vi "Exclude Zero Noise.vi"(7 "Counter in":dbl, 9 "RBF Weights in":dbl[](array[numeric]), 11 "RBF Weights previous in":dbl[](array[numeric])) -> (2 "RBF Weights out":dbl[](array[numeric]), 5 "Counter out":dbl)   [LabVIEW 2021]
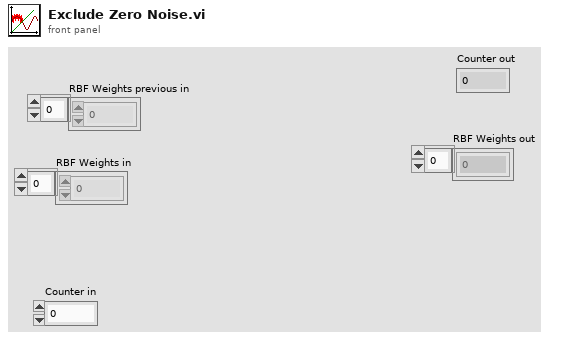
[diagram p1: front panel]
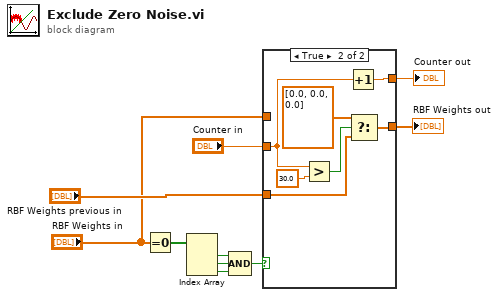
[diagram p0: block diagram]
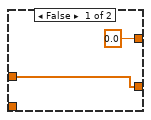
[diagram p2: hidden frame]
diagram:
  n1 = Equal To 0?(x="RBF Weights in") -> (x = 0?=w10:bool[])
  n2 = Index Array(array=w10) -> (element #1=w9:bool, element #2=w8:bool, element #3=w7:bool)  [unwired: 3 in]
  n3 = Compound Arithmetic op=AND(w9, w8, w7) -> (w6:bool)
  n4 = case shown="True" w6 {
    tunnel: "Counter in" -> [_ w17]
    tunnel: [0.0 w19] -> w4
    tunnel: [w11 w14] -> w3
    tunnel: "RBF Weights previous in" -> [_ w13]
    tunnel: "RBF Weights in" -> [w11 _]
    frame False {
    }
    frame True {
      n5 = Greater?(x=w17, y=30.0) -> (0:w16:bool)
      n6 = Increment(x=w17) -> (x+1=w19:dbl)
      n7 = Select(t=dbl[] [0.0, 0.0, 0.0], s=w16, f=w13) -> (s? t:f=w14:dbl[])
    }
  }
  "Counter out" <- w4
  "RBF Weights out" <- w3
